vi "inference_client.vi"() -> ()   [LabVIEW 2024]
uses:
  <vilib>/httpClient/POSTBuffer.vi
  <vilib>/httpClient/LabVIEWHTTPClient.lvlib
panel:
  out "concatenated string":string
  out "body":string
  out "headers":string
  out "data_path_string":string
  out "Application Directory":path
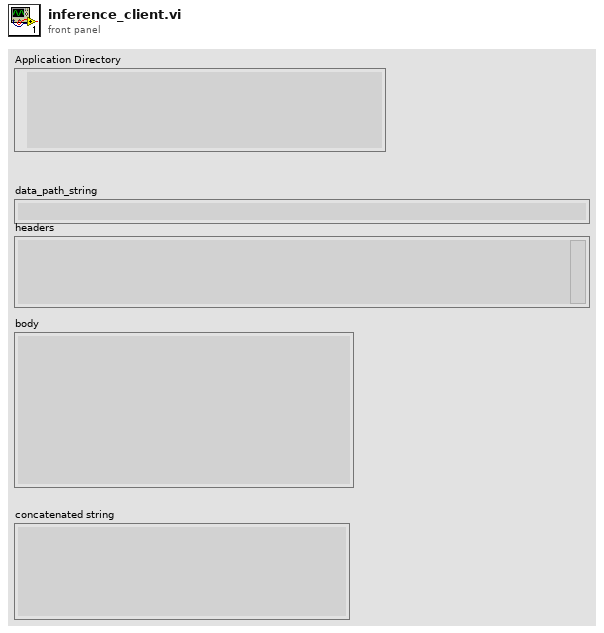
[diagram p1: front panel]
types:
  T1 = typedef "LabVIEWHTTPClient.lvlib/ClientHandle.ctl" = refnum<k1>
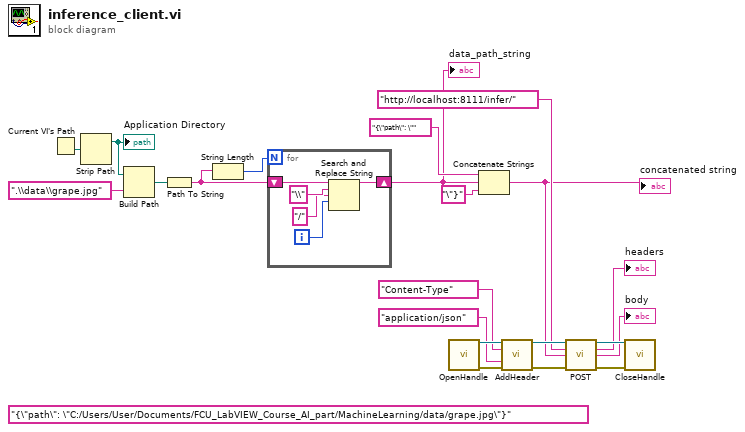
[diagram p0: block diagram]
diagram:
  (unwired) "{\"path\": \"C:/Users/User/Documents/FCU_LabVIEW_Course_AI_part/MachineLearning/data/grape.jpg\"}" ("buffer")
  n1 = Current VI's Path() -> (path=w2:path)
  n2 = Strip Path(path=w2) -> (stripped path=w1:path)  [unwired: 1 out]
  "Application Directory" <- w1
  n3 = Build Path(base path=w1, name or relative path=".\\data\\grape.jpg") -> (appended path=w20:path)
  n4 = Path To String(path=w20) -> (string=w18:string)
  n5 = String Length(string=w18) -> (length=w19:i32)
  n6 = for {
    N: w19 -> [_]
    shift-right: [w22] -> w4
    shift-left: w18 -> [w25]
    i -> [w23]
    n7 = Search and Replace String(input string=w25, search string="\\", replace string="/" ("replace string (\"\")"), offset=w23) -> (result string=w22:string)  [unwired: 4 in, 3 out]
  }
  "data_path_string" <- w4
  n8 = call <vilib>:"OpenHandle.vi"() -> ("client handle out"=w13:T1, "error out"=w12:errorcluster)  [unwired: 14 in]
  n9 = Concatenate Strings("{\"path\": \"" ("string"), w4, "\"}" ("string")) -> (w3:string)
  "concatenated string" <- w3
  n10 = call <vilib>:"AddHeader.vi"("client handle"=w13, "header"="Content-Type", "value"="application/json", "error in (no error)"=w12) -> ("client handle out"=w11:T1, "error out"=w10:errorcluster)  [unwired: 10 in]
  n11 = call-poly <vilib>:"POST.vi"("client handle"=w11, "url"="http://localhost:8111/infer/", "buffer"=w3, "error in (no error)"=w10) -> ("client handle out"=w17:T1, "headers"=→"headers":string, "body"=→"body":string, "error out"=w16:errorcluster)  [unwired: 8 in]
  n12 = call <vilib>:"CloseHandle.vi"("client handle"=w17, "error in (no error)"=w16) -> ()  [unwired: 13 in, 1 out]
